vi "StripURL.vi"(11 "URL":string) -> (2 "DataName":string, 3 "parentURL":string)   [LabVIEW 2017, in "TagDB.lvlib"]
uses:
  TagDB.lvlib
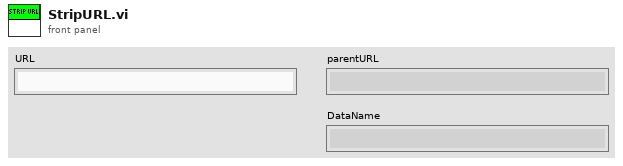
[diagram p1: front panel]
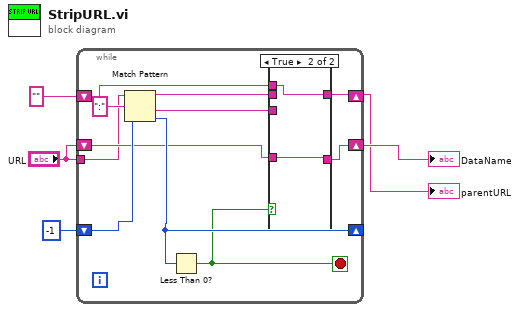
[diagram p0: block diagram]
diagram:
  n1 = while {
    shift-right: [w14] -> _
    shift-left: -1 -> [w15]
    shift-right: [w11] -> w4
    shift-left: "URL" -> [w12]
    shift-right: [w9] -> w3
    shift-left: "" -> [w7]
    tunnel: "URL" -> [w6]
    stop <- w13 stop-if-true
    n2 = Match Pattern(string=w6, regular expression=":", offset (0)=w15) -> (before substring=w8:string, after substring=w10:string, offset past match=w14:i32)  [unwired: 1 out]
    n3 = Less Than 0?(x=w14) -> (x < 0?=w13:bool)
    n4 = case shown="True" w13 {
      tunnel: w12 -> [_ w20]
      tunnel: [w18 w20] -> w11
      tunnel: w10 -> [w18 _]
      tunnel: [w17 w19] -> w9
      tunnel: w8 -> [w17 _]
      tunnel: w7 -> [_ w19]
      frame False {
      }
      frame True {
      }
    }
  }
  "parentURL" <- w3
  "DataName" <- w4
